vi "Request Data JSON.vi"(8 "error in (no error)":errorcluster, 11 "GetInputSettings in":refnum<class "GetInputSettings.lvclass">) -> (0 "error out":errorcluster, 2 "Request Data JSON":string, 3 "GetInputSettings out":refnum<class "GetInputSettings.lvclass">)   [LabVIEW 2020, in "obs-websocket.lvlib" / "GetInputSettings.lvclass"]
uses:
  GetInputSettings.lvclass
  GetInputSettings.lvclass/GetInputSettings.ctl
  a39a643b-14c7-4136-a2eb-584f84cc70a8.vi
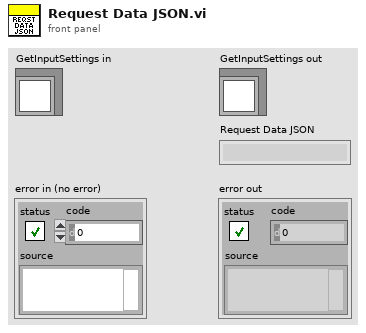
[diagram p1: front panel]
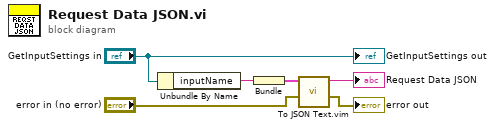
[diagram p0: block diagram]
diagram:
  n1 = Unbundle By Name("GetInputSettings in") -> ("inputName"=w5:string)
  n2 = Bundle("inputName"=w5) -> (w4:cluster{"inputName":string})  [unwired: 1 in]
  n3 = call "To JSON Text.vim"("error in (no error)"="error in (no error)", "Anything"=w4) -> ("error out"=→"error out":errorcluster, "<JSON>"=→"Request Data JSON":string)  [unwired: 8 in]
  "GetInputSettings out" <- "GetInputSettings in"
